vi "Finish.vi"   [LabVIEW 2017]
doc: "This VI is called just before exiting. It is expected to close I/O refnum, save collected data, etc."
uses:
  Utility VIs/Refnum Names.vi
  <vilib>/Rock Robotics/WPI/Utilities/WPI_GetSetVariantRefNum.vi
  Drive/Drive Globals.vi
  Intake/Intake Globals.vi
  Lift/Lift Globals.vi
  RPED/RPED Globals.vi
  Intake Rotation/Intake Rotation Globals.vi
  LEDs/LED Globals.vi
  <vilib>/Rock Robotics/Network Tables/NT Read Boolean.vi
  <vilib>/Rock Robotics/Network Tables/NT Write String.vi
types:
  T1 = typedef "WPI_DigitalInputDevRef.ctl" = cluster{"DevStatus":errorcluster, "DIO Channel":T2}
  T2 = typedef "FPGA_DIOChannel.ctl" = enum8{"DIO 0", "DIO 1", "DIO 2", "DIO 3", "DIO 4", "DIO 5", "DIO 6", "DIO 7", "DIO 8", "DIO 9", "DIO MXP 0", "DIO MXP 1", "DIO MXP 2", "DIO MXP 3", "DIO MXP 4", "DIO MXP 5", "DIO MXP 6", "DIO MXP 7", "DIO MXP 8", "DIO MXP 9", "DIO MXP 10", "DIO MXP 11", "DIO MXP 12", "DIO MXP 13", "DIO MXP 14", "DIO MXP 15", "SPI Port CS1", "SPI Port CS2", "SPI Port CS3", "SPI Port MISO", "SPI Port MOSI", "Invalid"}
  T3 = typedef "WPI_JoystickDevRef.ctl" = cluster{"Device":T4}
  T4 = typedef "WPI_JoystickDeviceEnum.ctl" = enum16{"USB 0", "USB 1", "USB 2", "USB 3", "USB 4", "USB 5"}
  T5 = typedef "WPI_SwitchDevRef.ctl" = cluster{"DevStatus":errorcluster, "DIO Channel":T2, "CntIndex":T6, "Normally Closed":bool}
  T6 = typedef "FPGA_CounterCtrSystemIndex.ctl" = enum8{"Ctr 0", "Ctr 1", "Ctr 2", "Ctr 3", "Ctr 4", "Ctr 5", "Ctr 6", "Ctr 7", "Invalid"}
  T7 = typedef "WPI_SolenoidDevRef.ctl" = cluster{"DevStatus":errorcluster, "Pneumatics Control Module":u8, "Forward Solenoid Channel":T8, "Reverse Solenoid Channel":T8}
  T8 = typedef "WPI_SolenoidChannel.ctl" = enum8{"Solenoid 0", "Solenoid 1", "Solenoid 2", "Solenoid 3", "Solenoid 4", "Solenoid 5", "Solenoid 6", "Solenoid 7", "Invalid"}
  T9 = typedef "WPI_MotorControlDeviceRef.ctl" = cluster{"DeviceStatus":errorcluster, "Type":T10, "PWM":cluster{"PWM Channel":T11, "DeadBand":T12}, "CAN":cluster{"Device Number":u8, "SetOutput VI Ref":variant, "GetOutput VI Ref":variant, "Enable VI Ref":variant, "Disable VI Ref":variant, "Data":variant}, "Invert":bool, "DIO PWM":cluster{"PWM \"Enable\" Channel":T11, "DIOChannel":T2, "PWM Rate":dbl}}
  T10 = typedef "WPI_MotorControlType.ctl" = enum16{"PWM", "CAN", "DIO PWM"}
  T11 = typedef "FPGA_DIOPWMChannel.ctl" = enum8{"PWM 0", "PWM 1", "PWM 2", "PWM 3", "PWM 4", "PWM 5", "PWM 6", "PWM 7", "PWM 8", "PWM 9", "PWM MXP 0", "PWM MXP 1", "PWM MXP 2", "PWM MXP 3", "PWM MXP 4", "PWM MXP 5", "PWM MXP 6", "PWM MXP 7", "PWM MXP 8", "PWM MXP 9", "Invalid"}
  T12 = typedef "WPI_PWMDeadband.ctl" = cluster{"Name":string, "maxPositivePwm":i32, "minPositivePwm":i32, "centerPwm":i32, "maxNegativePwm":i32, "minNegativePwm":i32, "angularRange":u16}
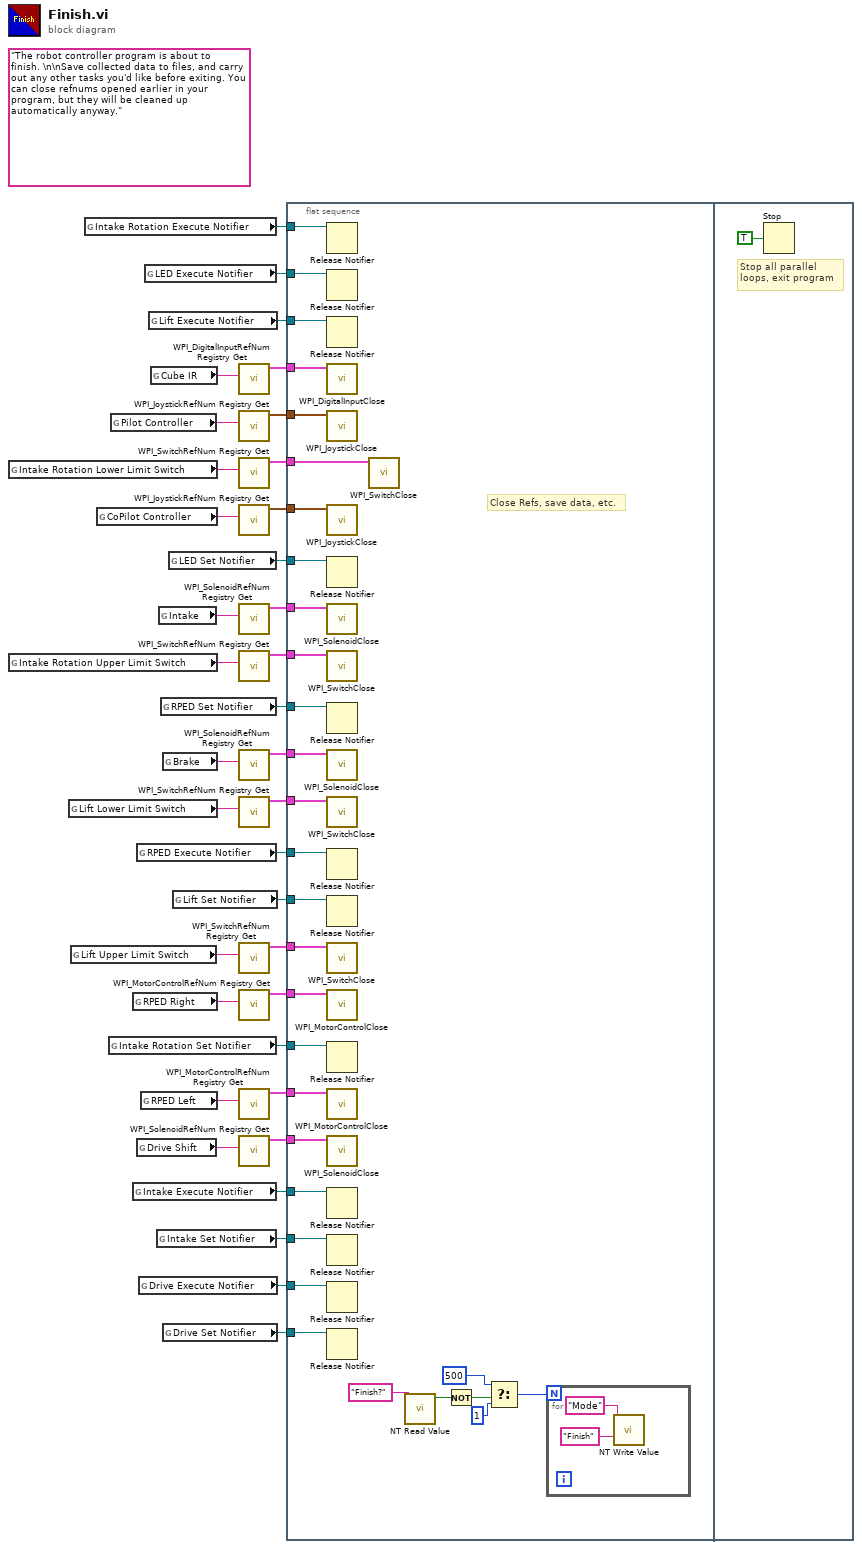
[diagram p0: block diagram]
diagram:
  (unwired) "The robot controller program is about to finish. \n\nSave collected data to files, and carry out any other tasks you'd like before exiting. You can close refnums opened earlier in your program, but they will be cleaned up automatically anyway."
  n1 = global read "Refnum Names.vi" "Intake Rotation Lower Limit Switch"() -> (w28:string)
  n2 = global read "Refnum Names.vi" "Intake Rotation Upper Limit Switch"() -> (w27:string)
  n3 = global read "Refnum Names.vi" "Lift Lower Limit Switch"() -> (w29:string)
  n4 = global read "Refnum Names.vi" "Lift Upper Limit Switch"() -> (w30:string)
  n5 = global read "Intake Rotation Globals.vi" "Intake Rotation Execute Notifier"() -> (w8:refnum<notifier>)
  n6 = global read "Refnum Names.vi" "CoPilot Controller"() -> (w34:string)
  n7 = global read "Intake Rotation Globals.vi" "Intake Rotation Set Notifier"() -> (w14:refnum<notifier>)
  n8 = global read "Refnum Names.vi" "Pilot Controller"() -> (w35:string)
  n9 = global read "Refnum Names.vi" "RPED Right"() -> (w2:string)
  n10 = global read "Intake Globals.vi" "Intake Execute Notifier"() -> (w9:refnum<notifier>)
  n11 = global read "RPED Globals.vi" "RPED Execute Notifier"() -> (w6:refnum<notifier>)
  n12 = global read "Refnum Names.vi" "Drive Shift"() -> (w18:string)
  n13 = global read "Drive Globals.vi" "Drive Execute Notifier"() -> (w10:refnum<notifier>)
  n14 = global read "Refnum Names.vi" "RPED Left"() -> (w1:string)
  n15 = global read "LED Globals.vi" "LED Execute Notifier"() -> (w5:refnum<notifier>)
  n16 = global read "Lift Globals.vi" "Lift Execute Notifier"() -> (w7:refnum<notifier>)
  n17 = global read "Refnum Names.vi" "Cube IR"() -> (w23:string)
  n18 = global read "Intake Globals.vi" "Intake Set Notifier"() -> (w15:refnum<notifier>)
  n19 = global read "Refnum Names.vi" "Intake"() -> (w20:string)
  n20 = global read "RPED Globals.vi" "RPED Set Notifier"() -> (w12:refnum<notifier>)
  n21 = global read "Refnum Names.vi" "Brake"() -> (w21:string)
  n22 = global read "Drive Globals.vi" "Drive Set Notifier"() -> (w16:refnum<notifier>)
  n23 = global read "LED Globals.vi" "LED Set Notifier"() -> (w11:refnum<notifier>)
  n24 = global read "Lift Globals.vi" "Lift Set Notifier"() -> (w13:refnum<notifier>)
  n25 = call <vilib>:"WPI_DigitalInputRefNum Registry Get.vi"("refnum name"=w23) -> ("DigitalInputDevRef"=w24:T1)  [unwired: 9 in, 1 out]
  n26 = call <vilib>:"WPI_JoystickRefNum Registry Get.vi"("refnum name"=w35) -> ("JoystickDevRef"=w36:T3)  [unwired: 9 in, 1 out]
  n27 = call <vilib>:"WPI_SwitchRefNum Registry Get.vi"("refnum name"=w28) -> ("SwitchDevRef"=w25:T5)  [unwired: 9 in, 1 out]
  n28 = call <vilib>:"WPI_JoystickRefNum Registry Get.vi"("refnum name"=w34) -> ("JoystickDevRef"=w33:T3)  [unwired: 9 in, 1 out]
  n29 = call <vilib>:"WPI_SolenoidRefNum Registry Get.vi"("refnum name"=w20) -> ("SolenoidDevRef"=w19:T7)  [unwired: 9 in, 1 out]
  n30 = call <vilib>:"WPI_SwitchRefNum Registry Get.vi"("refnum name"=w27) -> ("SwitchDevRef"=w26:T5)  [unwired: 9 in, 1 out]
  n31 = call <vilib>:"WPI_SolenoidRefNum Registry Get.vi"("refnum name"=w21) -> ("SolenoidDevRef"=w22:T7)  [unwired: 9 in, 1 out]
  n32 = call <vilib>:"WPI_SwitchRefNum Registry Get.vi"("refnum name"=w29) -> ("SwitchDevRef"=w31:T5)  [unwired: 9 in, 1 out]
  n33 = call <vilib>:"WPI_SwitchRefNum Registry Get.vi"("refnum name"=w30) -> ("SwitchDevRef"=w32:T5)  [unwired: 9 in, 1 out]
  n34 = call <vilib>:"WPI_MotorControlRefNum Registry Get.vi"("refnum name"=w2) -> ("MotorControlDevRef"=w4:T9)  [unwired: 9 in, 1 out]
  n35 = call <vilib>:"WPI_MotorControlRefNum Registry Get.vi"("refnum name"=w1) -> ("MotorControlDevRef"=w3:T9)  [unwired: 9 in, 1 out]
  n36 = call <vilib>:"WPI_SolenoidRefNum Registry Get.vi"("refnum name"=w18) -> ("SolenoidDevRef"=w17:T7)  [unwired: 9 in, 1 out]
  n37 = flat-sequence {
    tunnel: w36 -> [w66]
    tunnel: w33 -> [w65]
    tunnel: w32 -> [w64]
    tunnel: w31 -> [w63]
    tunnel: w26 -> [w62]
    tunnel: w25 -> [w61]
    tunnel: w24 -> [w60]
    tunnel: w22 -> [w59]
    tunnel: w19 -> [w58]
    tunnel: w17 -> [w57]
    tunnel: w16 -> [w56]
    tunnel: w15 -> [w55]
    tunnel: w14 -> [w54]
    tunnel: w13 -> [w53]
    tunnel: w12 -> [w52]
    tunnel: w11 -> [w51]
    tunnel: w10 -> [w50]
    tunnel: w9 -> [w49]
    tunnel: w8 -> [w48]
    tunnel: w7 -> [w47]
    tunnel: w6 -> [w46]
    tunnel: w5 -> [w45]
    tunnel: w4 -> [w44]
    tunnel: w3 -> [w43]
    frame #0 {
      # "Close Refs, save data, etc."
      n38 = Release Notifier(notifier=w48) -> ()  [unwired: 2 in, 3 out]
      n39 = Release Notifier(notifier=w45) -> ()  [unwired: 2 in, 3 out]
      n40 = Release Notifier(notifier=w47) -> ()  [unwired: 2 in, 3 out]
      n41 = call <vilib>:"WPI_DigitalInputClose.vi"("DigitalInputDevRef"=w60) -> ()  [unwired: 10 in, 1 out]
      n42 = call <vilib>:"WPI_JoystickClose.vi"("JoystickDevRef"=w66) -> ()  [unwired: 11 in]
      n43 = call <vilib>:"WPI_JoystickClose.vi"("JoystickDevRef"=w65) -> ()  [unwired: 11 in]
      n44 = Release Notifier(notifier=w51) -> ()  [unwired: 2 in, 3 out]
      n45 = call <vilib>:"WPI_SolenoidClose.vi"("SolenoidDevRef"=w58) -> ()  [unwired: 10 in, 1 out]
      n46 = call <vilib>:"WPI_SwitchClose.vi"("SwitchDevRef"=w62) -> ()  [unwired: 10 in, 1 out]
      n47 = Release Notifier(notifier=w52) -> ()  [unwired: 2 in, 3 out]
      n48 = call <vilib>:"WPI_SolenoidClose.vi"("SolenoidDevRef"=w59) -> ()  [unwired: 10 in, 1 out]
      n49 = call <vilib>:"WPI_SwitchClose.vi"("SwitchDevRef"=w63) -> ()  [unwired: 10 in, 1 out]
      n50 = Release Notifier(notifier=w46) -> ()  [unwired: 2 in, 3 out]
      n51 = Release Notifier(notifier=w53) -> ()  [unwired: 2 in, 3 out]
      n52 = call <vilib>:"WPI_SwitchClose.vi"("SwitchDevRef"=w64) -> ()  [unwired: 10 in, 1 out]
      n53 = call <vilib>:"WPI_MotorControlClose.vi"("MotorControlDevRef"=w44) -> ()  [unwired: 10 in, 1 out]
      n54 = Release Notifier(notifier=w54) -> ()  [unwired: 2 in, 3 out]
      n55 = call <vilib>:"WPI_MotorControlClose.vi"("MotorControlDevRef"=w43) -> ()  [unwired: 10 in, 1 out]
      n56 = call <vilib>:"WPI_SolenoidClose.vi"("SolenoidDevRef"=w57) -> ()  [unwired: 10 in, 1 out]
      n57 = Release Notifier(notifier=w49) -> ()  [unwired: 2 in, 3 out]
      n58 = Release Notifier(notifier=w55) -> ()  [unwired: 2 in, 3 out]
      n59 = Release Notifier(notifier=w50) -> ()  [unwired: 2 in, 3 out]
      n60 = Release Notifier(notifier=w56) -> ()  [unwired: 2 in, 3 out]
      n61 = call <vilib>:"WPI_SwitchClose.vi"("SwitchDevRef"=w61) -> ()  [unwired: 10 in, 1 out]
      n62 = call-poly <vilib>:"NT Read Value.vi"("Name"="Finish?") -> ("Boolean"=w40:bool)  [unwired: 9 in, 1 out]
      n63 = Not(x=w40) -> (.not. x?=w38:bool)
      n64 = Select(t=500, s=w38, f=1) -> (s? t:f=w41:i32)
      n65 = for {
        N: w41 -> [_]
        n66 = call-poly <vilib>:"NT Write Value.vi"("String"="Finish", "Name"="Mode") -> ()  [unwired: 9 in, 1 out]
      }
    }
    frame #1 {
      # "Stop all parallel\nloops, exit program"
      n67 = Stop(stop? (T)=TRUE ("Quit")) -> ()
    }
  }
